vi "Msg.vi"(7 "Actor in":refnum<class "Actor.lvclass">, 11 "Go To Destroy Msg in":refnum<class "Go To Destroy Msg.lvclass">) -> (0 "Error out":errorcluster, 5 "Actor out":refnum<class "Actor.lvclass">)   [LabVIEW 2020, in "jettl.lvlib" / "Go To Destroy Msg.lvlib" / "Go To Destroy Msg.lvclass"]
uses:
  Go To Destroy Msg.lvclass
  Actor/Actor/Actor.lvclass
  Go To Destroy/Go To Destroy.lvclass
  Go To Destroy Msg.lvclass/Go To Destroy Msg.ctl
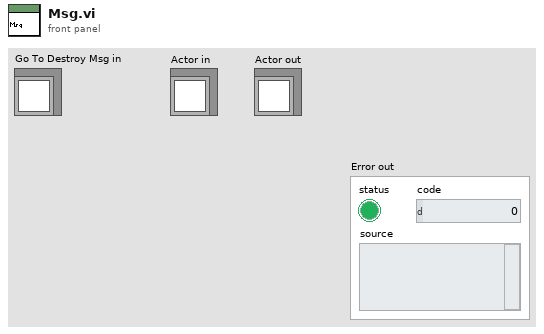
[diagram p1: front panel]
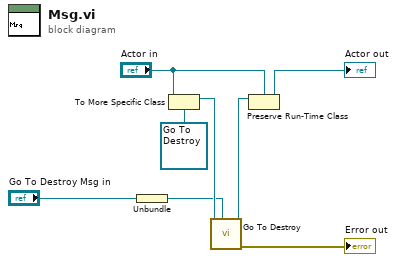
[diagram p0: block diagram]
diagram:
  n1 = Unbundle "Unbundle"("Go To Destroy Msg in") -> (w2:refnum<class "Sender.lvclass">)
  n2 = To More Specific Class(target class=refnum<class "Go To Destroy.lvclass"> refnum ("Destroy.lvlib:Destroy.lvclass"), reference="Actor in") -> (specific class reference=w4:refnum<class "Go To Destroy.lvclass">)  [unwired: 1 in, 1 out]
  n3 = call-dynamic "Go To Destroy.vi"("Sender"=w2, "Go To Destroy in"=w4) -> ("Error out"=→"Error out":errorcluster, "Go To Destroy out"=w3:refnum<class "Go To Destroy.lvclass">)  [unwired: 8 in]
  n4 = Preserve Run-Time Class(object in=w3, 2:"Actor in") -> (object out=→"Actor out":refnum<class "Actor.lvclass">)  [unwired: 1 in, 1 out]
